vi "create.watchlist.vi"(11 "watch.list":string[](array[string])=["AAPL"]) -> (3 "memory.config":u64[](array[numeric]) format="%.0x")   [LabVIEW 2022 SP3]
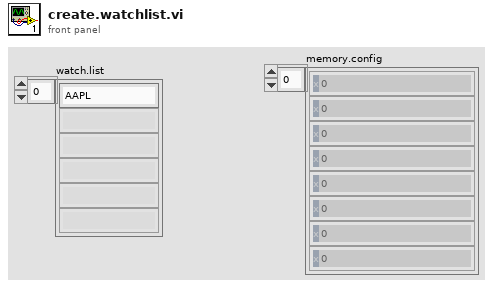
[diagram p1: front panel]
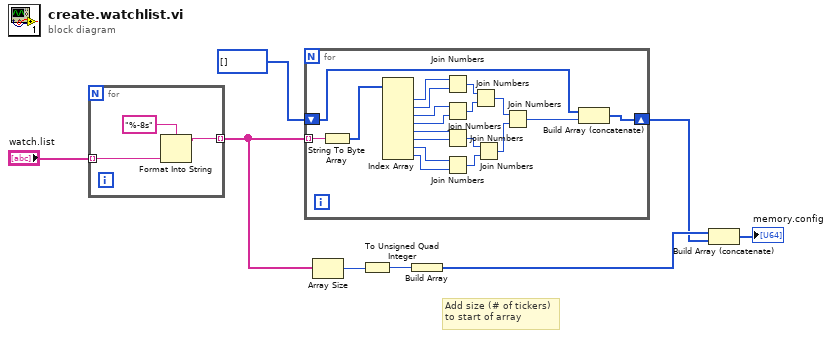
[diagram p0: block diagram]
diagram:
  # "Add size (# of tickers)\nto start of array"
  n1 = for {
    tunnel: "watch.list" -> [w10] mode=indexing
    tunnel: [w9] -> w5 mode=indexing
    n2 = Format Into String(format string="%-8s", w10) -> (resulting string=w9:string)  [unwired: 2 in, 1 out]
  }
  n3 = for {
    tunnel: w5 -> [w30] mode=indexing
    shift-right: [w14] -> w1
    shift-left: u64[] [] -> [w12]
    n4 = String To Byte Array(string=w30) -> (unsigned byte array=w29:u8[])
    n5 = Index Array(array=w29) -> (element #1=w28:u8, element #2=w27:u8, element #3=w26:u8, element #4=w25:u8, element #5=w24:u8, element #6=w23:u8, element #7=w22:u8, element #8=w21:u8)  [unwired: 8 in]
    n6 = Join Numbers(hi=w28, lo=w27) -> ((hi.lo)=w20:u16)
    n7 = Join Numbers(hi=w26, lo=w25) -> ((hi.lo)=w19:u16)
    n8 = Join Numbers(hi=w24, lo=w23) -> ((hi.lo)=w18:u16)
    n9 = Join Numbers(hi=w22, lo=w21) -> ((hi.lo)=w17:u16)
    n10 = Join Numbers(hi=w20, lo=w19) -> ((hi.lo)=w16:u32)
    n11 = Join Numbers(hi=w18, lo=w17) -> ((hi.lo)=w15:u32)
    n12 = Join Numbers(hi=w16, lo=w15) -> ((hi.lo)=w13:u64)
    n13 = Build Array (concatenate)(w12, w13) -> (w14:u64[])
  }
  n14 = Array Size(array=w5) -> (size(s)=w6:i32)
  n15 = To Unsigned Quad Integer(1:w6) -> (0:w8:u64)
  n16 = Build Array(w8) -> (w4:u64[])
  n17 = Build Array (concatenate)(w4, w1) -> (→"memory.config":u64[])
